vi "Send simple mesage.vi"(4 "Content":variant, 7 "Sender":string, 8 "error in (no error)":errorcluster, 11 "Mailbox ref in":T1) -> (0 "error out":errorcluster, 2 "timed out?":bool, 3 "mailbox ref out":T1)   [LabVIEW 2021, in "MatS Libs.lvlib"]
doc: "Puts simple message into mailbox.\nSimple message contains info about: sender, content, and timestamp with current time."
uses:
  <userlib>/MatS Libs/MatS Mailman/TypeDefs/Mailbox ref.ctl
  <userlib>/MatS Libs/MatS Mailman/TypeDefs/Simple message.ctl
  <userlib>/MatS Libs/MatS Libs.lvlib
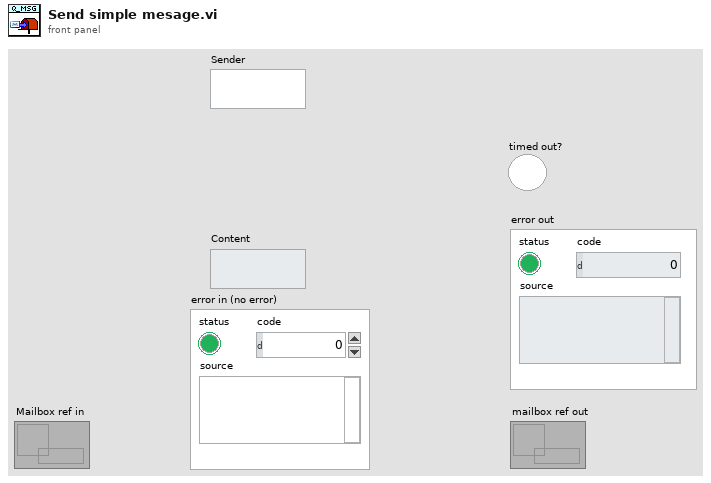
[diagram p1: front panel]
types:
  T1 = typedef "MatS Libs.lvlib/Mailbox ref.ctl" = refnum<queue>
  T2 = typedef "MatS Libs.lvlib/Simple message.ctl" = cluster{"Sender":string, "Content":variant, "Timestamp":timestamp}
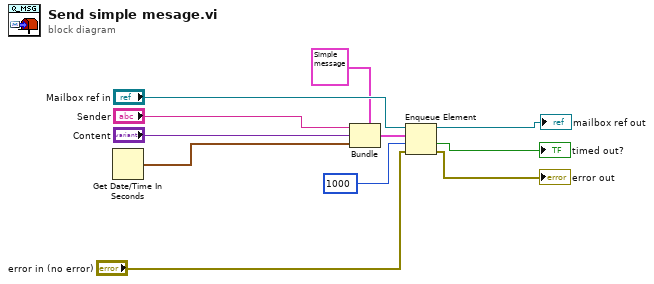
[diagram p0: block diagram]
diagram:
  n1 = Get Date/Time In Seconds() -> (seconds since 1Jan1904=w8:timestamp)
  n2 = Bundle(cluster=T2 {"Sender"="", "Content"=variant, "Timestamp"=timestamp(0 s since 1904-01-01)}, "Sender"="Sender", "Content"="Content", "Timestamp"=w8) -> (w7:T2)
  n3 = Enqueue Element(queue="Mailbox ref in", element=w7, timeout in ms (-1)=1000, error in (no error)="error in (no error)") -> (queue out=→"mailbox ref out":T1, timed out?=→"timed out?":bool, error out=→"error out":errorcluster)
